vi "niDTS WLAN INSTR TX Configure Hardware.vi"(8 "error in (no error)":errorcluster, 11 "niDTS WLAN INSTR TX in":refnum<class "niDTS WLAN INSTR TX.lvclass">) -> (0 "error out":errorcluster, 3 "niDTS WLAN INSTR TX out":refnum<class "niDTS WLAN INSTR TX.lvclass">)   [LabVIEW 2015, in "niDTS WLAN.lvlib" / "niDTS WLAN INSTR TX.lvclass"]
doc: "Sets:\n\n* AcquisitionLengthMode\n* AcquisitionLengthDuration\n* AutoLevelEnabled"
uses:
  niDTS WLAN INSTR TX.lvclass
  niDTS WLAN INSTR TX.lvclass/niDTS WLAN INSTR TX.ctl
  RiviInstDriver/niRfsaWlan/Objects/niRfsaWlan.lvclass
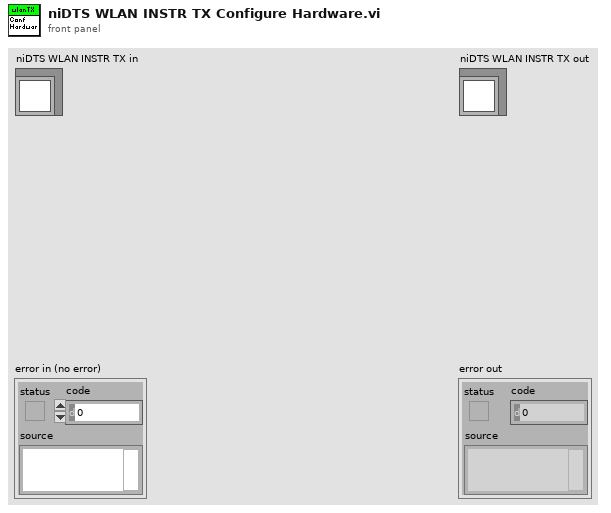
[diagram p1: front panel]
types:
  T1 = typedef "niRfsaWlan.lvclass/niRfsaWlan INC Handle.ctl" = refnum<data-value>
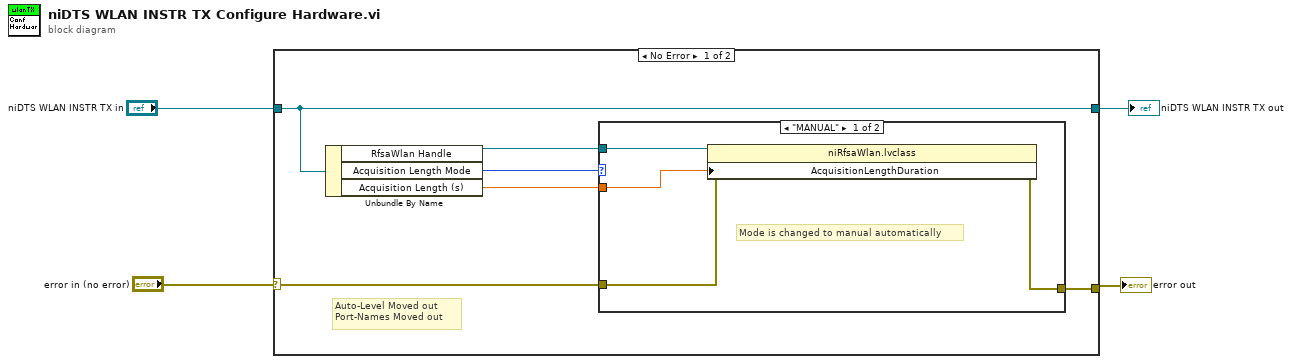
[diagram p0: block diagram]
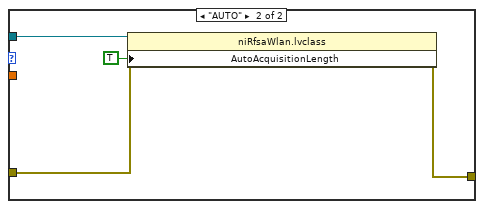
[diagram p2: hidden frame]
diagram:
  n1 = case shown="No Error" "error in (no error)" {
    selector: "error in (no error)" -> [w8 w20]
    tunnel: [w7 w20] -> w3
    tunnel: [w9 w19] -> w1
    tunnel: "niDTS WLAN INSTR TX in" -> [w9 w19]
    frame No Error {
      # "Auto-Level Moved out\nPort-Names Moved out"
      n2 = Unbundle By Name(w9) -> ("RfsaWlan Handle"=w10:T1, "Acquisition Length Mode"=w5:enum16{"AUTO", "MANUAL"}, "Acquisition Length (s)"=w6:dbl)
      n3 = case shown="\"MANUAL\"" w5 {
        tunnel: w10 -> [w14 w18]
        tunnel: w8 -> [w13 w17]
        tunnel: [w12 w16] -> w7
        tunnel: w6 -> [w11 _]
        frame "MANUAL" {
          # "Mode is changed to manual automatically"
          n4 = property class="niRfsaWlan.lvclass"(reference=w14, error in=w13, "AcquisitionLengthDuration"=w11) -> (error out=w12:errorcluster)  [unwired: 1 out]
        }
        frame "AUTO" {
          n5 = property class="niRfsaWlan.lvclass"(reference=w18, error in=w17, "AutoAcquisitionLength"=TRUE ("CONFigure:RFSA:WLAN:ALENgth:AutoAcquisitionLength")) -> (error out=w16:errorcluster)  [unwired: 1 out]
        }
      }
    }
    frame Error {
    }
  }
  "error out" <- w3
  "niDTS WLAN INSTR TX out" <- w1
